vi "Divide Amplitude and Offset by Output Gain.vi"(8 "error in (no error)":errorcluster, 11 "Instrument.DAQ":refnum<class "Instrument.DAQ.lvclass">) -> (0 "error out":errorcluster, 3 "Instrument.DAQ out":refnum<class "Instrument.DAQ.lvclass">)   [LabVIEW 2019, in "Instrument.Lockin.lvlib" / "Instrument.DAQ.lvclass"]
uses:
  Instrument.DAQ.lvclass
  Instrument.DAQ.lvclass/Instrument.DAQ.ctl
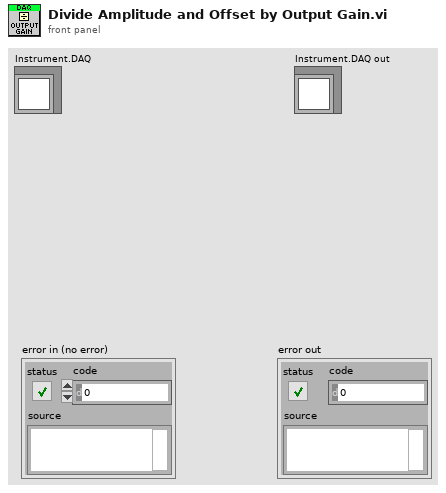
[diagram p1: front panel]
types:
  T1 = typedef "Instrument.Lockin.lvlib/Instrument.DAQ.lvclass/AO.Channel--Cluster--Array.ctl" = T2[]
  T2 = typedef "Instrument.Lockin.lvlib/Instrument.DAQ.lvclass/AO.Channel--Cluster.ctl" = cluster{"Enable?":bool, "Channel":i32, "Amplitude":dbl, "Offset":dbl, "Frequency":dbl, "Phase":dbl, "Function":T3, "Sweeping?":bool, "Limit AC":bool, "Limit DC?":bool, "Duty Cycle":bool}
  T3 = typedef "Instrument.Lockin.lvlib/Instrument.DAQ.lvclass/AO.Channel.Function--Enum.ctl" = enum16{"sine", "square", "triangle", "saw"}
  T4 = typedef "Instrument.Lockin.lvlib/Instrument.DAQ.lvclass/Channel.Gain--Cluster--Array.ctl" = T5[]
  T5 = typedef "Instrument.Lockin.lvlib/Instrument.DAQ.lvclass/Channel.Gain--Cluster.ctl" = cluster{"Channel":string, "Gain":dbl}
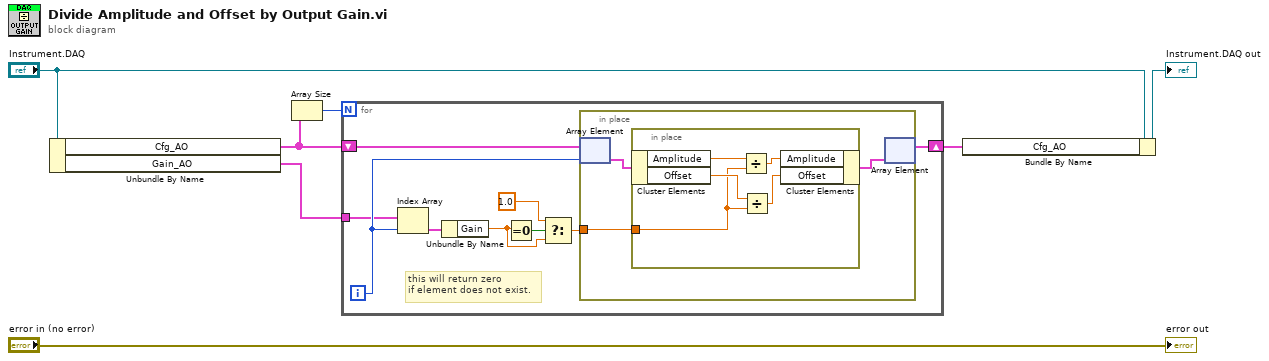
[diagram p0: block diagram]
diagram:
  n1 = Unbundle By Name("Instrument.DAQ") -> ("Cfg_AO"=w5:T1, "Gain_AO"=w1:T4)
  n2 = Array Size(array=w5) -> (size(s)=w6:i32)
  n3 = for {
    N: w6 -> [_]
    tunnel: w1 -> [w11]
    shift-right: [w16] -> w2
    shift-left: w5 -> [w14]
    i -> [w15]
    # "this will return zero\nif element does not exist."
    n4 = Index Array(array=w11, index=w15) -> (element=w9:T5)
    n5 = Unbundle By Name(w9) -> ("Gain"=w8:dbl)
    n6 = Equal To 0?(x=w8) -> (x = 0?=w13:bool)
    n7 = Select(t=1.0, s=w13, f=w8) -> (s? t:f=w10:dbl)
    n8 = in-place {
      in-place-border: w10 -> [w19]
      n9 = in-place-array #1(w14, w15) -> (w17:T2)
      n10 = in-place {
        in-place-border: w19 -> [w21]
        n11 = in-place-cluster #2(w17) -> ("Amplitude"=w24:dbl, "Offset"=w22:dbl)
        n12 = Divide(x=w24, y=w21) -> (x/y=w23:dbl)
        n13 = Divide(x=w22, y=w21) -> (x/y=w20:dbl)
        n14 = in-place-cluster #2("Amplitude"=w23, "Offset"=w20) -> (w18:T2)
      }
      n15 = in-place-array #1(w18) -> (w16:T1)  [unwired: 1 out]
    }
  }
  n16 = Bundle By Name(cluster="Instrument.DAQ", "Cfg_AO"=w2) -> (→"Instrument.DAQ out":refnum<class "Instrument.DAQ.lvclass">)
  "error out" <- "error in (no error)"
